vi "BlockDiagram_CreateDiagram.vi"(7 "PythonConverter in":refnum<class "PythonBDConverter.lvclass">, 8 "error in":errorcluster, 11 "VI Interpreter in":refnum<class "VI Interpreter.lvclass">) -> (0 "error out":errorcluster, 3 "VI Interpreter out":refnum<class "VI Interpreter.lvclass">, 4 "create_diagram":string, 5 "PythonConverter out":refnum<class "PythonBDConverter.lvclass">)   [LabVIEW 2014, in "PythonBDConverter.lvclass"]
uses:
  PythonBDConverter.lvclass
  VI Interpreter/Classes/VI Interpreter/VI Interpreter.lvclass
  Parsing/ClassTypeTD.ctl
  VI Interpreter/Classes/TopLevelDiagram/TopLevelDiagram.lvclass
  Parsing/Python Functions.lvlib
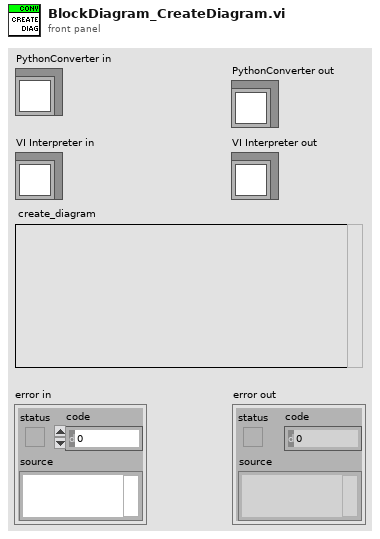
[diagram p1: front panel]
types:
  T1 = typedef "Python Functions.lvlib/ClassTypeTD.ctl" = enum16{"class", "function"}
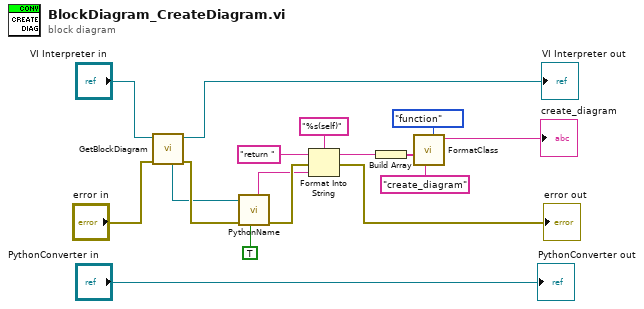
[diagram p0: block diagram]
diagram:
  n1 = call "GetBlockDiagram.vi"("error in"="error in", "VI Interpreter in"="VI Interpreter in") -> ("error out"=w5:errorcluster, "VI Interpreter out"=→"VI Interpreter out":refnum<class "VI Interpreter.lvclass">, "TopLevelDiagram"=w4:refnum<class "TopLevelDiagram.lvclass">)  [unwired: 5 in]
  n2 = call-dynamic "PythonName.vi"("add self"=TRUE, "error in"=w5, "Diagram in"=w4) -> ("error out"=w10:errorcluster, "name"=w8:string)  [unwired: 5 in, 2 out]
  n3 = Format Into String(format string="%s(self)", initial string="return ", error in=w10, w8) -> (resulting string=w7:string, error out=→"error out":errorcluster)
  n4 = Build Array(w7) -> (w2:string[])
  n5 = call "FormatClass.vi"("type"=ClassTypeTD."function", "name"="create_diagram", "body"=w2) -> ("python"=→"create_diagram":string)  [unwired: 8 in]
  "PythonConverter out" <- "PythonConverter in"
